vi "Read Ranges.vi"(8 "error in (no error)":errorcluster, 11 "FormulaG API in":refnum<class "FormulaG API.lvclass">) -> (0 "error out":errorcluster, 2 "Ranges":T1, 3 "FormulaG API out":refnum<class "FormulaG API.lvclass">)   [LabVIEW 2020, in "FormulaG.lvlib" / "FormulaG API.lvclass"]
uses:
  FormulaG API.lvclass
  FormulaLV-Common/Ranges.ctl
  Command.ctl
  FormulaG API.lvclass/FormulaG API.ctl
  <vilib>/IlluminatedG/lv-stream/stream/Stream.lvclass/Stream.ctl
  <vilib>/IlluminatedG/lv-stream/stream/Dispatch Sniffer Data.vi
  <vilib>/IlluminatedG/lv-stream/stream/Prepared.vi
  <vilib>/IlluminatedG/lv-stream/Endpoint/Cast Sniffer Callback.vi
  <vilib>/IlluminatedG/IG WebSocket Stream/Stream-Websocket/WebsocketStream/WebsocketStream.lvclass
  C:/Program Files (x86)/National Instruments/LabVIEW 2020/vi.lib/IlluminatedG/lv-stream/stream/Stream.lvclass
  <vilib>/Utility/error.llb/Error Cluster From Error Code.vi
  <vilib>/IlluminatedG/lv-stream/stream/Stream.lvclass
  FormulaLV-Common/FormulaG-Common.lvlib
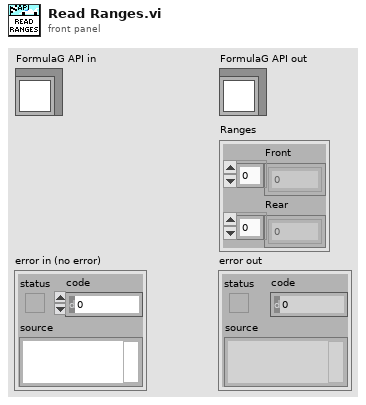
[diagram p1: front panel]
types:
  T1 = typedef "FormulaG-Common.lvlib/Ranges.ctl" = cluster{"Front":sgl[], "Rear":sgl[]}
  T2 = enum16{"big-endian, network order", "native, host order", "little-endian"}
  T3 = typedef "FormulaG.lvlib/FormulaG API.lvclass/Command.ctl" = enum8{"None", "Reset Car", "Request Ranges", "Control Car", "Request Info", "Set Options", "Set Camera", "Set Pause"}
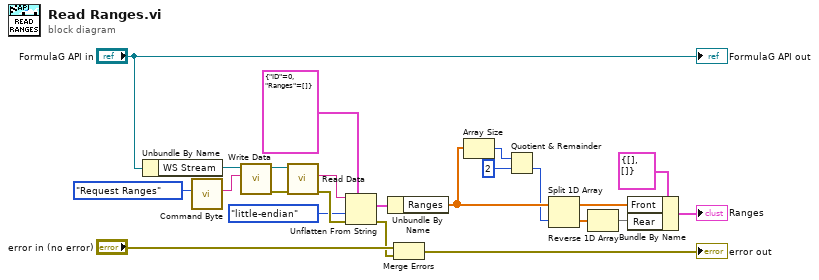
[diagram p0: block diagram]
diagram:
  n1 = Unbundle By Name("FormulaG API in") -> ("WS Stream"=w16:refnum<class "WebsocketStream.lvclass">)
  n2 = call "Command Byte.vi"("Command"=Command."Request Ranges") -> ("Command Byte"=w15:string)  [unwired: 10 in]
  n3 = call <vilib>:"Write Data.vi"("Data"=w15, "Stream in"=w16) -> ("error out"=w12:errorcluster, "Stream out"=w19:refnum<class "WebsocketStream.lvclass">)  [unwired: 8 in]
  n4 = call <vilib>:"Read Data.vi"("error in (no error)"=w12, "Stream in"=w19) -> ("error out"=w23:errorcluster, "Data"=w18:string)  [unwired: 7 in, 1 out]
  n5 = Unflatten From String(type=cluster{"ID":u8, "Ranges":sgl[]} {"ID"=0, "Ranges"=[]}, binary string=w18, byte order (0:big-endian, network order)=T2."little-endian", error in (no error)=w23) -> (value=w13:cluster{"ID":u8, "Ranges":sgl[]}, error out=w6:errorcluster)  [unwired: 1 in, 1 out]
  n6 = Unbundle By Name(w13) -> ("Ranges"=w9:sgl[])
  n7 = Merge Errors("error in (no error)", w6) -> (→"error out":errorcluster)
  n8 = Array Size(array=w9) -> (size(s)=w11:i32)
  n9 = Quotient & Remainder(x=w11, y=2) -> (floor(x/y)=w8:i32)  [unwired: 1 out]
  n10 = Split 1D Array(array=w9, index=w8) -> (first subarray=w2:sgl[], second subarray=w3:sgl[])
  n11 = Reverse 1D Array(array=w3) -> (reversed array=w1:sgl[])
  n12 = Bundle By Name(cluster=T1 {"Front"=[], "Rear"=[]} ("Ranges"), "Front"=w2, "Rear"=w1) -> (→"Ranges":T1)
  "FormulaG API out" <- "FormulaG API in"
